vi "Wait.vi"(4 "error in":errorcluster caption="error out", 6 "Zu wartende ms":u32=250, 7 "VISA resource name in":refnum<visa-resource-name>) -> (0 "error out":errorcluster, 3 "VISA resource name out":refnum<visa-resource-name>)   [LabVIEW 2015, in "JULABO DeviceDriver.lvlib"]
uses:
  JULABO DeviceDriver.lvlib
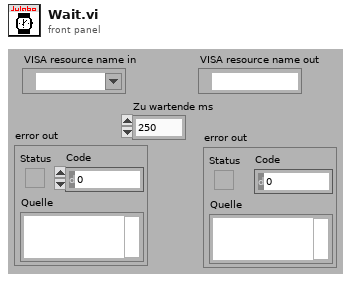
[diagram p1: front panel]
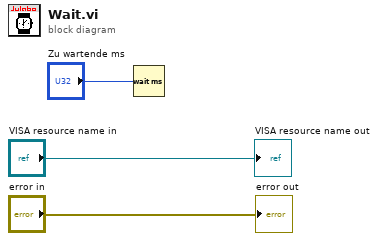
[diagram p0: block diagram]
diagram:
  n1 = Wait (ms)(milliseconds to wait="Zu wartende ms") -> ()  [unwired: 1 out]
  "VISA resource name out" <- "VISA resource name in"
  "error out" <- "error in"
